vi "Datasheet No Preview.vi"(8 "error in":errorcluster, 10 "sxTemplateId":string, 11 "Paths":T1[](array[typedef])) -> (0 "error out":errorcluster, 3 "Array":T1[](array[typedef]))   [LabVIEW 2011]
uses:
  Datasheet Report Info.ctl
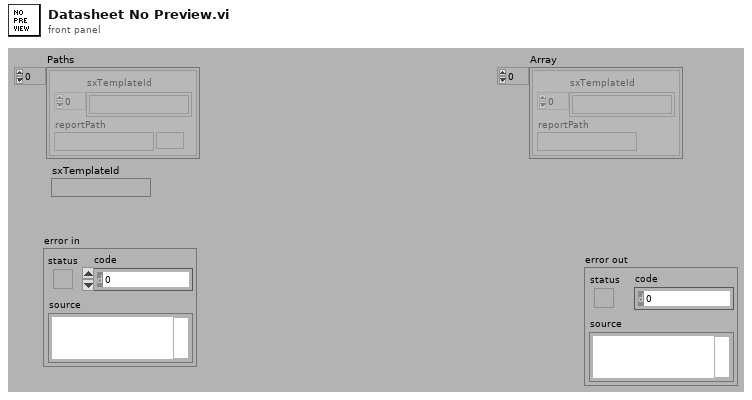
[diagram p1: front panel]
types:
  T1 = typedef "Datasheet Report Info.ctl" = cluster{"sxTemplateId":string[], "reportPath":path}
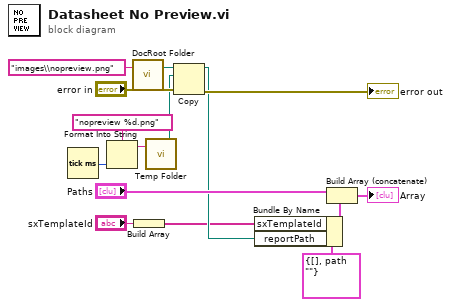
[diagram p0: block diagram]
diagram:
  n1 = Tick Count (ms)() -> (millisecond timer value=w9:u32)
  n2 = Format Into String(format string="nopreview %d.png" ("name or relative path"), w9) -> (resulting string=w10:string)  [unwired: 2 in, 1 out]
  n3 = call "DocRoot Folder.vi"("Relative Path (\"\" - Folder)"="images\\nopreview.png" ("name or relative path")) -> ("DocumentRoot Folder"=w1:path)  [unwired: 2 in]
  n4 = Build Array("sxTemplateId") -> (w3:string[])
  n5 = call "Temp Folder.vi"("Relative Path (\"\")"=w10) -> ("Temp Folder"=w11:path)  [unwired: 2 in]
  n6 = Copy(8:"error in", 10:w11, 11:w1) -> (0:→"error out":errorcluster, 3:w5:path)  [unwired: 3 out]
  n7 = Bundle By Name(cluster=T1 {"sxTemplateId"=[], "reportPath"=path ""} ("report"), "sxTemplateId"=w3, "reportPath"=w5) -> (w6:T1)
  n8 = Build Array (concatenate)("Paths", w6) -> (→"Array":T1[])
